vi "ConnectDevice.vi"(8 "Error in":errorcluster, 11 "Devices":refnum<k24>[](array[refnum])) -> (0 "Error out":errorcluster, 2 "Result":bool, 3 "Devices":refnum<k24>[](array[refnum]))   [LabVIEW 2016]
doc: "Connects all given devices.\n\nDevices: Array of devices to connect\nResult: True if no warning or error occurred during connect"
uses:
  C:/Users/CL/Desktop/ZcDAQprj0811/ZcDAQprj/Modules/DAQ-Device/Hardware Drivers/QX/HBM LabVIEW Driver/DLLs/Hbm.Api.Common.dll
  DLLs/Hbm.Api.Common.dll
  C:/Users/CL/Desktop/ZcDAQprj0811/ZcDAQprj/Modules/DAQ-Device/Hardware Drivers/QX/HBM LabVIEW Driver/DLLs/Hbm.Api.LabVIEW.dll
  DLLs/Hbm.Api.LabVIEW.dll
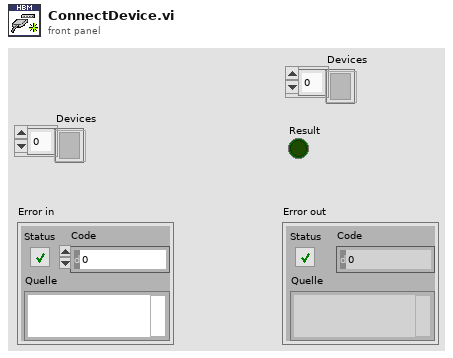
[diagram p1: front panel]
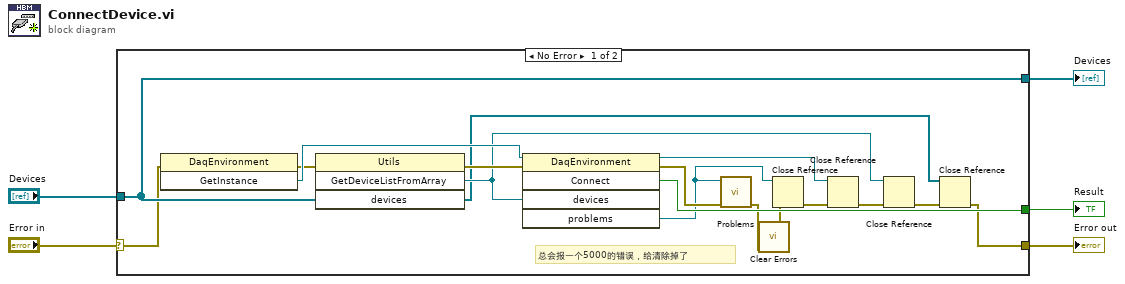
[diagram p0: block diagram]
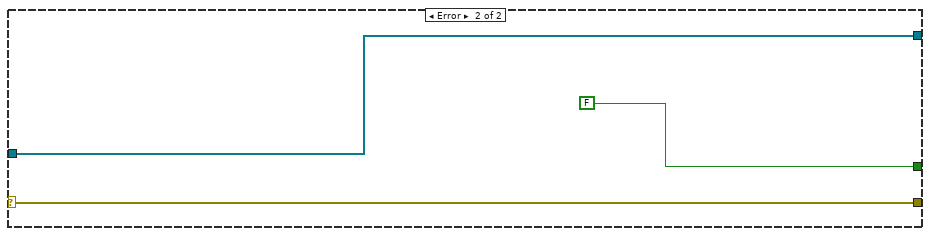
[diagram p2: hidden frame]
diagram:
  n1 = case shown="No Error" "Error in" {
    selector: "Error in" -> [w18 w25]
    tunnel: [w8 w25] -> w4
    tunnel: [w22 FALSE ("Connect")] -> w3
    tunnel: "Devices" -> [w19 w24]
    tunnel: [w19 w24] -> w1
    frame No Error {
      # "总会报一个5000的错误，给清除掉了"
      n2 = invoke on="Methodenknoten" class="DaqEnvironment" method="GetInstance"(error in=w18) -> (error out=w16:errorcluster, "GetInstance"=w17:refnum<k24>)  [unwired: 2 in, 1 out]
      n3 = invoke on="Methodenknoten" class="Utils" method="GetDeviceListFromArray"(error in=w16, "devices"=w19) -> (error out=w21:errorcluster, "GetDeviceListFromArray"=w10:refnum<k24>, "devices"=w7:refnum<k24>[])  [unwired: 2 in, 1 out]
      n4 = invoke class="DaqEnvironment" method="Connect"(reference=w17, error in=w21, "devices"=w10) -> (reference out=w15:refnum<k24>, error out=w20:errorcluster, "Connect"=w22:bool, "problems"=w12:refnum<k24>)  [unwired: 2 in, 1 out]
      n5 = call "Problems.vi"("Error in"=w20, "Problems"=w12) -> ("Error out"=w13:errorcluster)  [unwired: 9 in]
      n6 = call <vilib>:"Clear Errors.vi"("error in (no error)"=w13) -> ("error out"=w6:errorcluster)  [unwired: 5 in, 1 out]
      n7 = Close Reference(reference=w12, error in (no error)=w6) -> (error out=w14:errorcluster)
      n8 = Close Reference(reference=w15, error in (no error)=w14) -> (error out=w11:errorcluster)
      n9 = Close Reference(reference=w10, error in (no error)=w11) -> (error out=w9:errorcluster)
      n10 = Close Reference(reference=w7, error in (no error)=w9) -> (error out=w8:errorcluster)
    }
    frame Error {
    }
  }
  "Error out" <- w4
  "Result" <- w3
  "Devices" <- w1
